vi "Search Tree Path.vi"(8 "Error In":errorcluster, 10 "Tree Path":string, 11 "Tree Manager":refnum<data-value>) -> (0 "Error Out":errorcluster, 3 "Tree Manager":refnum<data-value>, 5 "Tree IDs":string[](array[string]))   [LabVIEW 2017, in "Tree API.lvlib" / "Tree.lvclass"]
doc: "Search by using the specified Tree Path. The Tree Path should contain a sequence of names, each index specifying another level. The syntax should mimic a web URL with / symbols between levels. If the Tree ID is wired in it will be used as the base of the search.\n\nExample: Parent/Nested1/Nested2/Nested3 corresponds to a Tree with 4 levels, each containing one Child Tree.\n\nThis search mechanism will return multiple Tree IDs if the search path had many matching results i.e. was complex."
uses:
  Tree.lvclass
  <vilib>/ErrorRing/Error Ring.xnode
  <vilib>/Utility/error.llb/Error Cluster From Error Code.vi
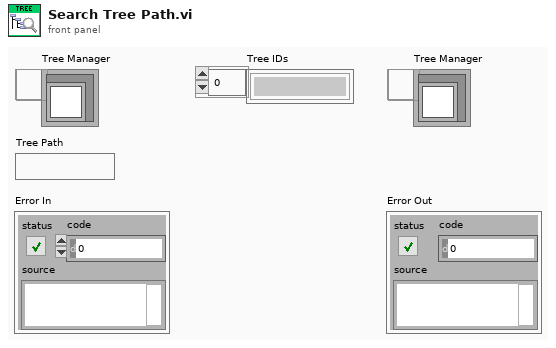
[diagram p1: front panel]
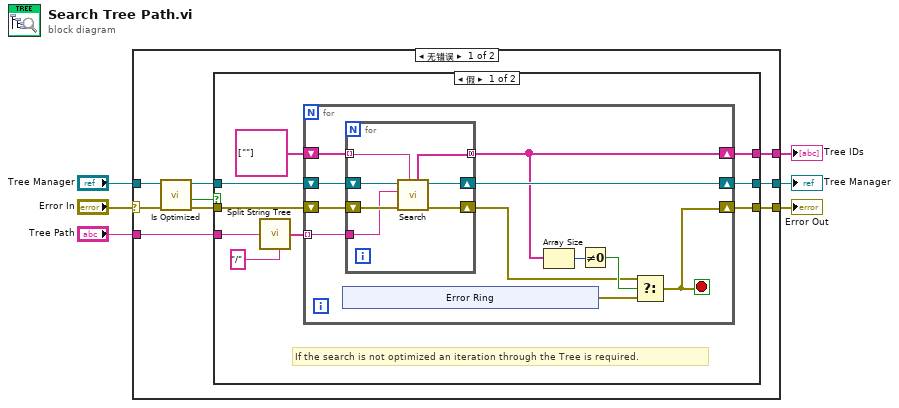
[diagram p0: block diagram]
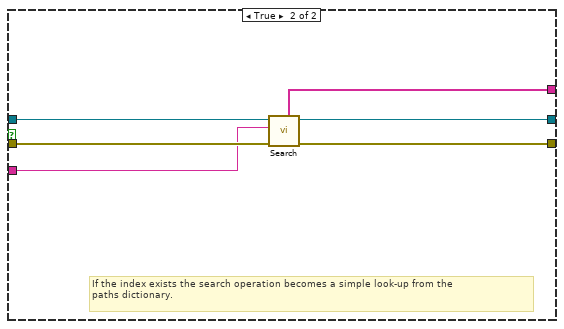
[diagram p2: hidden frame]
diagram:
  n1 = case shown="无错误" "Error In" {
    selector: "Error In" -> [w7 w54]
    tunnel: [w15 _] -> w6
    tunnel: [w14 w54] -> w5
    tunnel: [w13 w55] -> w4
    tunnel: "Tree Manager" -> [w12 w55]
    tunnel: "Tree Path" -> [w8 _]
    frame No Error {
      n2 = call "Is Optimized.vi"("Error In"=w7, "Tree Manager"=w12) -> ("Error Out"=w9:errorcluster, "Is Optimized?"=w10:bool, "Tree Manager"=w11:refnum<data-value>)  [unwired: 7 in]
      n3 = case shown="假" w10 {
        tunnel: [w24 w50] -> w15
        tunnel: [w23 w48] -> w14
        tunnel: [w22 w49] -> w13
        tunnel: w11 -> [w21 w53]
        tunnel: w9 -> [w20 w52]
        tunnel: w8 -> [w17 w51]
        frame False {
          # "If the search is not optimized an iteration through the Tree is required."
          n4 = call "Split String Tree.vi"("Split Pattern"="/", "Input String"=w17) -> ("Split String"=w18:string[])  [unwired: 5 in]
          n5 = for {
            shift-right: [w34] -> w22
            shift-left: w21 -> [w35]
            tunnel: w18 -> [w31] mode=indexing
            shift-right: [w30] -> w24
            shift-left: string[] [""] ("IDs") -> [w32]
            shift-right: [w25] -> w23
            shift-left: w20 -> [w33]
            stop <- w25 stop-if-true
            n6 = xnode "Error Ring"() -> ("错误输出"=w26:errorcluster)
            n7 = for {
              tunnel: w32 -> [w43] mode=indexing
              tunnel: w31 -> [w42]
              tunnel: [w41] -> w30 mode=concatenating
              shift-right: [w46] -> w34
              shift-left: w35 -> [w47]
              shift-right: [w44] -> w27
              shift-left: w33 -> [w45]
              n8 = call "Search.vi"("Parent ID"=w43, "Error In"=w45, "Name or Tree Path"=w42, "Tree Manager"=w47) -> ("Error Out"=w44:errorcluster, "Tree Manager"=w46:refnum<data-value>, "IDs"=w41:string[])  [unwired: 5 in]
            }
            n9 = Array Size(array=w30) -> (size(s)=w29:i32)
            n10 = Not Equal To 0?(x=w29) -> (x != 0?=w28:bool)
            n11 = Select(t=w27, s=w28, f=w26) -> (s? t:f=w25:errorcluster)
          }
        }
        frame True {
          # "If the index exists the search operation becomes a simple look-up from the\npaths dictionary."
          n12 = call "Search.vi"("Error In"=w52, "Name or Tree Path"=w51, "Tree Manager"=w53) -> ("Error Out"=w48:errorcluster, "Tree Manager"=w49:refnum<data-value>, "IDs"=w50:string[])  [unwired: 6 in]
        }
      }
    }
    frame Error {
    }
  }
  "Tree IDs" <- w6
  "Error Out" <- w5
  "Tree Manager" <- w4
